vi "Open Front Panel.vi"(8 "error in (no error)":errorcluster, 11 "VI Data in":refnum<class "VI Data.lvclass">) -> (0 "error out":errorcluster, 3 "VI Data out":refnum<class "VI Data.lvclass">)   [LabVIEW 2013, in "SET Project Data.lvlib" / "VI Data.lvclass"]
uses:
  VI Data.lvclass
  VI Data.lvclass/VI Data.ctl
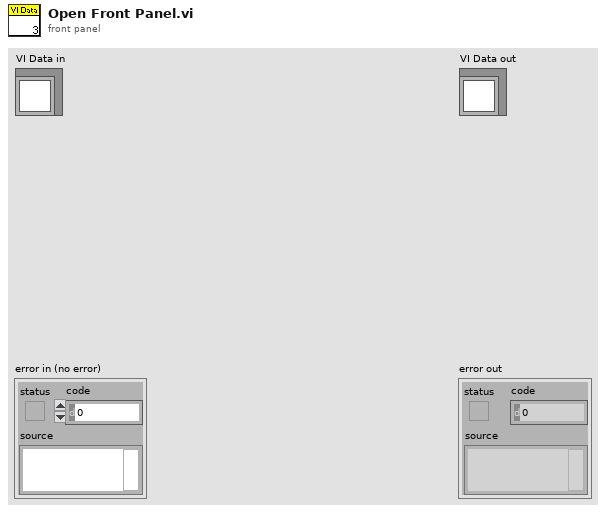
[diagram p1: front panel]
types:
  T1 = enum32{"Invalid", "Standard", "Closed", "Hidden", "Minimized", "Maximized"}
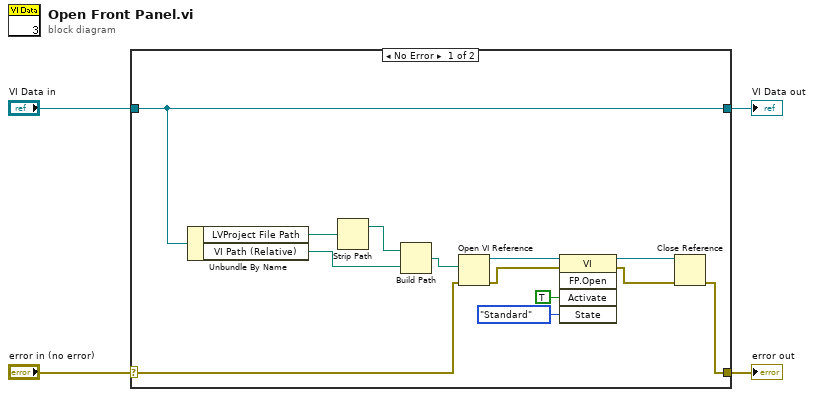
[diagram p0: block diagram]
diagram:
  n1 = case shown="No Error" "error in (no error)" {
    selector: "error in (no error)" -> [w12 w19]
    tunnel: [w5 w19] -> w3
    tunnel: [w13 w18] -> w1
    tunnel: "VI Data in" -> [w13 w18]
    frame No Error {
      n2 = Unbundle By Name(w13) -> ("LVProject File Path"=w17:path, "VI Path (Relative)"=w14:path)
      n3 = Strip Path(path=w17) -> (stripped path=w16:path)  [unwired: 1 out]
      n4 = Build Path(base path=w16, name or relative path=w14) -> (appended path=w15:path)
      n5 = Open VI Reference(vi path=w15, error in (no error)=w12) -> (vi reference=w11:refnum<vi>, error out=w8:errorcluster)  [unwired: 4 in]
      n6 = invoke class="VI" method="FP.Open"(reference=w11, error in=w8, "Activate"=TRUE ("Activate?"), "State"=T1."Standard") -> (reference out=w7:refnum<vi>, error out=w6:errorcluster)  [unwired: 1 in, 3 out]
      n7 = Close Reference(reference=w7, error in (no error)=w6) -> (error out=w5:errorcluster)
    }
    frame Error {
    }
  }
  "error out" <- w3
  "VI Data out" <- w1
